vi "PTPS.vi"() -> ()   [LabVIEW 2021]
uses:
  <vilib>/Utility/file.llb/Write Delimited Spreadsheet (string).vi
  <vilib>/Utility/file.llb/Write Delimited Spreadsheet (DBL).vi
panel:
  in  "Krok obliczeń":dbl=1.0 min=0.1 step=0.1
  in  "t":dbl=50.0
  in  "Rszcz = 0":bool
  in  "c2 = 0":bool
  in  "Robc = INF":bool
  in  "Rszcz":dbl=10.0
  in  "I2":dbl=200.0
  in  "U1":dbl=40.0
  in  "Robc":dbl=40.0
  out "Waveform Graph":waveform(dbl)(graph)={"t0"=timestamp(0 s since 1904-01-01), "dt"=1.0, "Y"=[0.0, 0.0, 0.0, 0.0, 0.0, 0.0, 0.0, 0.0, 0.0, 0.0, 1.9999999999999716, 3.9999999999999716, 5.999999999999972, 7.999999999999972, 9.999999999999972, 11.999999999999972, 13.999999999999972, 15.999999999999972, 17.99999999999997, 19.99999999999997, 21.99999999999997, 23.99999999999997, 25.99999999999997, 27.99999999999997, 29.99999999999997]}
  in  "R1":dbl=40.0
  in  "R2":dbl=50.0
  in  "L12":dbl=2.0 step=0.1
  in  "L2":dbl=50.0 step=0.1
  in  "Menu Ring":u16(ring)=1 items=["Stan ustalony", "Stan nieustalony inercyjny", "Stan nieustalony różniczkujący"]
  in  "Info Button":bool caption="Home Button"
  in  "Fi1":dbl=1000.0
  in  "c1":dbl=1.0
  in  "c2":dbl=1.0
  in  "wr":dbl=50.0
  in  "SWPS Button":bool caption="Home Button"
  in  "Exit Button":bool caption="Home Button"
  in  "Save Button":bool caption="Home Button"
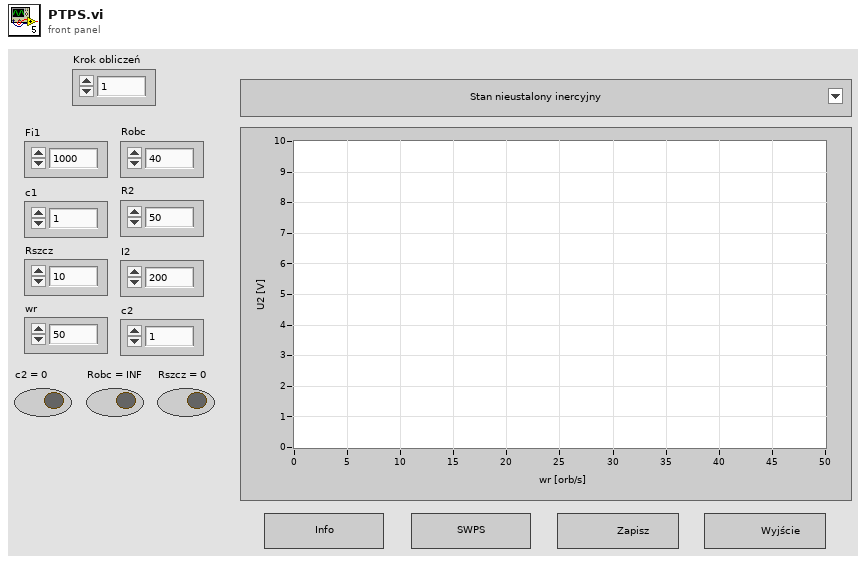
[diagram p1: front panel]
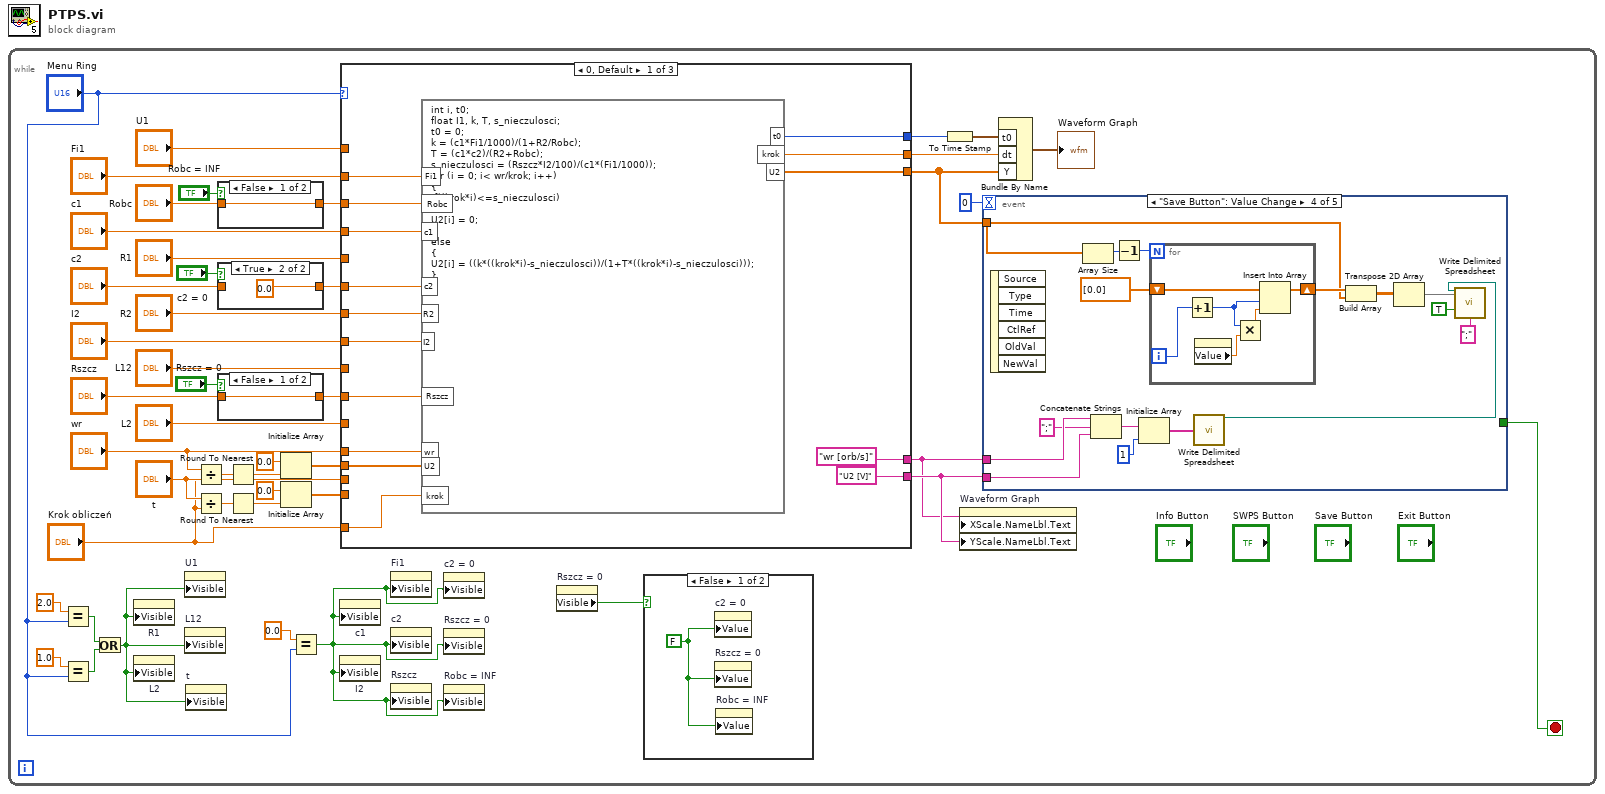
[diagram p0: block diagram]
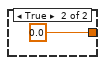
[diagram p4: hidden frame]
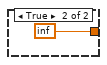
[diagram p5: hidden frame]
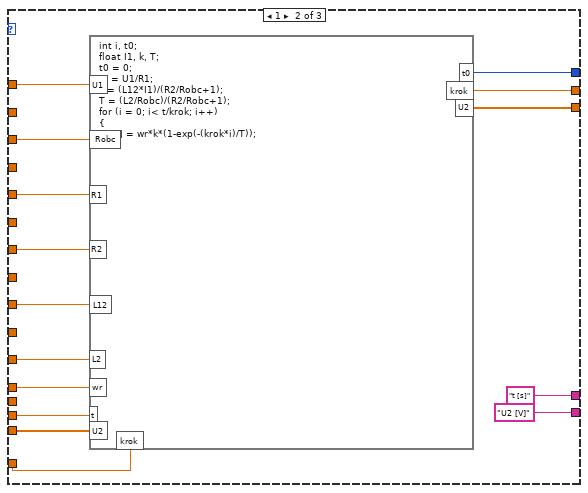
[diagram p6: hidden frame]
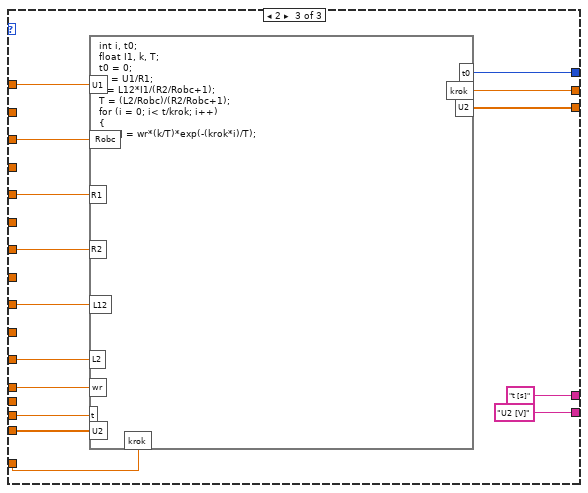
[diagram p7: hidden frame]
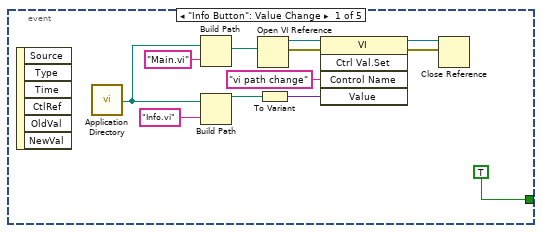
[diagram p8: hidden frame]
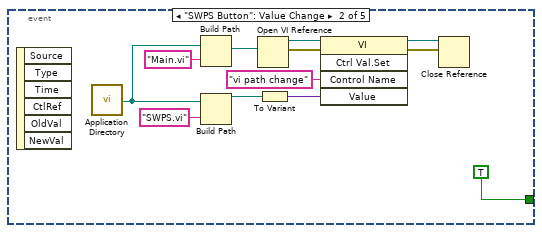
[diagram p9: hidden frame]
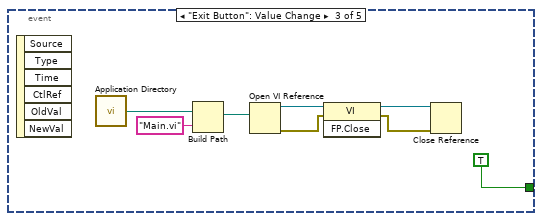
[diagram p10: hidden frame]
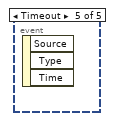
[diagram p11: hidden frame]
diagram:
  n1 = while {
    stop <- w38 stop-if-true
    n2 = Equal?(x=2.0, y="Menu Ring") -> (x = y?=w17:bool)
    n3 = Equal?(x=1.0, y="Menu Ring") -> (x = y?=w18:bool)
    n4 = Or(x=w17, y=w18) -> (x .or. y?=w12:bool)
    n5 = property on="R1" class="DigNum (strict)"("Visible"=w12) -> ()  [unwired: 2 in, 2 out]
    n6 = property on="L2" class="DigNum (strict)"("Visible"=w12) -> ()  [unwired: 2 in, 2 out]
    n7 = property on="U1" class="DigNum (strict)"("Visible"=w12) -> ()  [unwired: 2 in, 2 out]
    n8 = property on="L12" class="DigNum (strict)"("Visible"=w12) -> ()  [unwired: 2 in, 2 out]
    n9 = property on="t" class="DigNum (strict)"("Visible"=w12) -> ()  [unwired: 2 in, 2 out]
    n10 = Divide(x="wr", y="Krok obliczeń") -> (x/y=w5:dbl)
    n11 = Divide(x="t", y="Krok obliczeń") -> (x/y=w4:dbl)
    n12 = case shown="False" "Robc = INF" {
      tunnel: [w52 inf] -> w26
      tunnel: "Robc" -> [w52 _]
      frame False {
      }
      frame True {
      }
    }
    n13 = case shown="True" "c2 = 0" {
      tunnel: "c2" -> [w48 _]
      tunnel: [w48 0.0] -> w23
      frame False {
      }
      frame True {
      }
    }
    n14 = case shown="False" "Rszcz = 0" {
      tunnel: "Rszcz" -> [w50 _]
      tunnel: [w50 0.0] -> w19
      frame False {
      }
      frame True {
      }
    }
    n15 = Round To Nearest(number=w5) -> (nearest integer value=w6:dbl)
    n16 = Round To Nearest(number=w4) -> (nearest integer value=w7:dbl)
    n17 = Initialize Array(0.0 ("element"), w6) -> (w13:dbl[])
    n18 = Initialize Array(0.0 ("element"), w7) -> (w15:dbl[])
    n19 = Equal?(x=0.0, y="Menu Ring") -> (x = y?=w8:bool)
    n20 = property on="c1" class="DigNum (strict)"("Visible"=w8) -> ()  [unwired: 2 in, 2 out]
    n21 = property on="I2" class="DigNum (strict)"("Visible"=w8) -> ()  [unwired: 2 in, 2 out]
    n22 = case shown="0, Default" "Menu Ring" {
      tunnel: "U1" -> [_ w83 w98]
      tunnel: w26 -> [w68 w82 w97]
      tunnel: "R1" -> [_ w81 w96]
      tunnel: "R2" -> [w67 w80 w95]
      tunnel: "L12" -> [_ w79 w94]
      tunnel: "L2" -> [_ w78 w93]
      tunnel: [w66 w77 w92] -> w11
      tunnel: [w65 w76 w91] -> w32
      tunnel: [w55 w75 w90] -> w40
      tunnel: ["wr [orb/s]" "t [s]" "t [s]"] -> w33
      tunnel: ["U2 [V]" "U2 [V]" "U2 [V]"] -> w34
      tunnel: "Fi1" -> [w62 _ _]
      tunnel: "c1" -> [w61 _ _]
      tunnel: w23 -> [w60 _ _]
      tunnel: "I2" -> [w59 _ _]
      tunnel: w19 -> [w58 _ _]
      tunnel: "wr" -> [w57 w72 w87]
      tunnel: "t" -> [_ w71 w86]
      tunnel: w15 -> [_ w70 w85]
      tunnel: w13 -> [w56 _ _]
      tunnel: "Krok obliczeń" -> [w54 w69 w84]
      frame 0, Default {
        n23 = formula code="int i, t0;\nfloat I1, k, T, s_nieczulosci;\nt0 = 0;\nk = (c1*Fi1/1000)/(1+R2/Robc);\nT = (c1*c2)/(R2+Robc);\ns_nieczulosci = (Rszcz*I2/100)/(c1*(Fi1/1000));\nfor (i = 0; i< wr/krok; i++)\n{\nif((krok*i)<=s_nieczulosci)\n{\nU2[i] = 0;\n}\nelse\n{\nU2[i] = ((k*((krok*i)-s_nieczulosci))/(1+T*((krok*i)-s_nieczulosci)));\n}\n}"("Fi1"=w62, "Robc"=w68, "c1"=w61, "R2"=w67, "c2"=w60, "I2"=w59, "Rszcz"=w58, "wr"=w57, "U2"=w56, "krok"=w54) -> ("U2"=w66:dbl[], "krok"=w65:dbl, "t0"=w55:i32)
      }
      frame 1 {
        n24 = formula code="int i, t0;\nfloat I1, k, T;\nt0 = 0;\nI1 = U1/R1;\nk = (L12*I1)/(R2/Robc+1);\nT = (L2/Robc)/(R2/Robc+1);\nfor (i = 0; i< t/krok; i++)\n{\nU2[i] = wr*k*(1-exp(-(krok*i)/T));\n}"("U1"=w83, "Robc"=w82, "R1"=w81, "R2"=w80, "L12"=w79, "L2"=w78, "wr"=w72, "t"=w71, "U2"=w70, "krok"=w69) -> ("U2"=w77:dbl[], "krok"=w76:dbl, "t0"=w75:i32)
      }
      frame 2 {
        n25 = formula code="int i, t0;\nfloat I1, k, T;\nt0 = 0;\nI1 = U1/R1;\nk = L12*I1/(R2/Robc+1);\nT = (L2/Robc)/(R2/Robc+1);\nfor (i = 0; i< t/krok; i++)\n{\nU2[i] = wr*(k/T)*exp(-(krok*i)/T);\n}"("U1"=w98, "Robc"=w97, "R1"=w96, "R2"=w95, "L12"=w94, "L2"=w93, "wr"=w87, "t"=w86, "U2"=w85, "krok"=w84) -> ("U2"=w92:dbl[], "krok"=w91:dbl, "t0"=w90:i32)
      }
    }
    n26 = property on="Fi1" class="DigNum (strict)"("Visible"=w8) -> ()  [unwired: 2 in, 2 out]
    n27 = property on="c2" class="DigNum (strict)"("Visible"=w8) -> ()  [unwired: 2 in, 2 out]
    n28 = property on="Rszcz" class="DigNum (strict)"("Visible"=w8) -> ()  [unwired: 2 in, 2 out]
    n29 = property on="c2 = 0" class="Bool (strict)"("Visible"=w8) -> ()  [unwired: 2 in, 2 out]
    n30 = property on="Rszcz = 0" class="Bool (strict)"("Visible"=w8) -> ()  [unwired: 2 in, 2 out]
    n31 = property on="Robc = INF" class="Bool (strict)"("Visible"=w8) -> ()  [unwired: 2 in, 2 out]
    n32 = property on="Rszcz = 0" class="Bool (strict)"() -> ("Visible"=w9:bool)  [unwired: 2 in, 2 out]
    n33 = case shown="False" w9 {
      frame False {
        w47 = FALSE ("c2 = 0")
        n34 = property on="c2 = 0" class="Bool (strict)"("Value"=w47) -> ()  [unwired: 2 in, 2 out]
        n35 = property on="Rszcz = 0" class="Bool (strict)"("Value"=w47) -> ()  [unwired: 2 in, 2 out]
        n36 = property on="Robc = INF" class="Bool (strict)"("Value"=w47) -> ()  [unwired: 2 in, 2 out]
      }
      frame True {
      }
    }
    n37 = To Time Stamp(1:w40) -> (0:w41:timestamp)
    n38 = property on="Waveform Graph" class="WFGraph (strict)"("XScale.NameLbl.Text"=w33, "YScale.NameLbl.Text"=w34) -> ()  [unwired: 2 in, 2 out]
    n39 = event shown="[3] \"Save Button\": Value Change" {
      selector: _ -> [_ _ _ _ _]
      dyn-events: _ -> [_ _ _ _ _]
      timeout: 0 -> [_ _ _ _ _]
      tunnel: [TRUE TRUE TRUE _ _] -> w38
      tunnel: w34 -> [_ _ _ w136 _]
      tunnel: w33 -> [_ _ _ w135 _]
      tunnel: w11 -> [_ _ _ w145 _]
      event "Info Button": Value Change {
        n40 = event-data() -> ()  [unwired: 1 in, 6 out]
        n41 = call <vilib>:"Application Directory.vi"() -> ("Application Directory"=w100:path)
        n42 = Build Path(base path=w100, name or relative path="Main.vi") -> (appended path=w101:path)
        n43 = Build Path(base path=w100, name or relative path="Info.vi") -> (appended path=w103:path)
        n44 = Open VI Reference(vi path=w101) -> (vi reference=w108:refnum<vi>, error out=w109:errorcluster)  [unwired: 5 in]
        n45 = To Variant(anything=w103) -> (Variant=w110:variant)
        n46 = invoke class="VI" method="Ctrl Val.Set"(reference=w108, error in=w109, "Control Name"="vi path change", "Value"=w110) -> (reference out=w107:refnum<vi>, error out=w106:errorcluster)  [unwired: 1 in, 3 out]
        n47 = Close Reference(reference=w107, error in (no error)=w106) -> ()  [unwired: 1 out]
      }
      event "SWPS Button": Value Change {
        n48 = event-data() -> ()  [unwired: 1 in, 6 out]
        n49 = call <vilib>:"Application Directory.vi"() -> ("Application Directory"=w112:path)
        n50 = Build Path(base path=w112, name or relative path="Main.vi") -> (appended path=w113:path)
        n51 = Build Path(base path=w112, name or relative path="SWPS.vi") -> (appended path=w115:path)
        n52 = Open VI Reference(vi path=w113) -> (vi reference=w120:refnum<vi>, error out=w121:errorcluster)  [unwired: 5 in]
        n53 = To Variant(anything=w115) -> (Variant=w122:variant)
        n54 = invoke class="VI" method="Ctrl Val.Set"(reference=w120, error in=w121, "Control Name"="vi path change", "Value"=w122) -> (reference out=w119:refnum<vi>, error out=w118:errorcluster)  [unwired: 1 in, 3 out]
        n55 = Close Reference(reference=w119, error in (no error)=w118) -> ()  [unwired: 1 out]
      }
      event "Exit Button": Value Change {
        n56 = event-data() -> ()  [unwired: 1 in, 6 out]
        n57 = call <vilib>:"Application Directory.vi"() -> ("Application Directory"=w128:path)
        n58 = Build Path(base path=w128, name or relative path="Main.vi") -> (appended path=w129:path)
        n59 = Open VI Reference(vi path=w129) -> (vi reference=w126:refnum<vi>, error out=w124:errorcluster)  [unwired: 5 in]
        n60 = invoke class="VI" method="FP.Close"(reference=w126, error in=w124) -> (reference out=w125:refnum<vi>, error out=w123:errorcluster)  [unwired: 1 in, 1 out]
        n61 = Close Reference(reference=w125, error in (no error)=w123) -> ()  [unwired: 1 out]
      }
      event "Save Button": Value Change {
        n62 = event-data() -> ()  [unwired: 1 in, 6 out]
        n63 = Array Size(array=w145) -> (size(s)=w141:i32)
        n64 = Concatenate Strings(w135, ";" ("delimiter (\\t)"), w136) -> (w133:string)
        n65 = Decrement(x=w141) -> (x-1=w140:i32)
        n66 = Initialize Array(w133, 1 ("dimension size")) -> (w132:string[])
        n67 = for {
          N: w140 -> [_]
          shift-right: [w152] -> w146
          shift-left: dbl[] [0.0] -> [w151]
          i -> [w150]
          n68 = Increment(x=w150) -> (x+1=w147:i32)
          n69 = property on="Krok obliczeń" class="DigNum (strict)"() -> ("Value"=w149:dbl)  [unwired: 2 in, 2 out]
          n70 = Multiply(x=w147, y=w149) -> (x*y=w148:dbl)
          n71 = Insert Into Array(array=w151, index=w147, new element=w148) -> (w152:dbl[])
        }
        n72 = call-poly <vilib>:"Write Delimited Spreadsheet.vi"("1D data"=w132) -> ("new file path (Not A Path if cancelled)"=w143:path)  [unwired: 13 in, 1 out]
        n73 = Build Array(w146, w145) -> (w139:dbl[][])
        n74 = Transpose 2D Array(2D array=w139) -> (transposed array=w138:dbl[][])
        n75 = call-poly <vilib>:"Write Delimited Spreadsheet.vi"("file path (dialog if empty)"=w143, "2D data"=w138, "append to file? (new file:F)"=TRUE, "delimiter (\\t)"=";" ("delimiter (\\t)")) -> ()  [unwired: 10 in, 2 out]
      }
      event Timeout {
        n76 = event-data() -> ()  [unwired: 1 in, 3 out]
      }
    }
    n77 = Bundle By Name("t0"=w41, "dt"=w32, "Y"=w11) -> (→"Waveform Graph":waveform(dbl))  [unwired: 1 in]
  }
